vi "Sperre thrust alloc SF30K (SubVI) old.vi"(0 "Thruster rpms":dbl[](array[numeric]), 1 "manip14":u8, 2 "manip15":u8, 3 "manip16":u8, 5 "error in":errorcluster, 6 "dim 1+2":u8, 7 "Light 1":bool, 8 "dim 3+4":u8, 9 "Light 2":bool, 10 "digital2":u8, 11 "Light 3":bool, 12 "digital3":u8=2, 13 "Light 4":bool, 17 "HMI 1":bool, 18 "HMI 2":bool) -> (14 "telebuf":u8[](array[numeric]), 19 "error IO":errorcluster)   [LabVIEW 2011]
uses:
  <vilib>/imath/engines/lvmath2/RunTimeEngine/ErrorHandling/NIMS_Finalize Error.vi
  <vilib>/imath/engines/lvmath2/RunTimeEngine/BuiltInFunctions/uint8/NIMS_uint8(int).vi
  <instcachedir>/0/NIMS_uint8(int)_9D6EF81F86254677BB00410F9E5C6A1D.lvgen/NIMS_uint8(int)_9D6EF81F86254677BB00410F9E5C6A1D_000.vi
  <vilib>/imath/engines/lvmath2/RunTimeEngine/NodeEndStatement/NIMS_NodeEndStatement_Output.vi
  <instcachedir>/0/NIMS_NodeEndStatement_Output_53EC0D466D134D7ABD903AC30B43404B.lvgen/NIMS_NodeEndStatement_Output_53EC0D466D134D7ABD903AC30B43404B_016.vi
  <vilib>/imath/engines/lvmath2/RunTimeEngine/BuiltInFunctions/round/NIMS_round(DBL-S).vi
  <vilib>/imath/engines/lvmath2/RunTimeEngine/BuiltInFunctions/uint8/NIMS_uint8(real).vi
  <instcachedir>/0/NIMS_uint8(real)_CAA419FBB1354DA296C59E18C46DECF0.lvgen/NIMS_uint8(real)_CAA419FBB1354DA296C59E18C46DECF0_000.vi
  <instcachedir>/0/NIMS_uint8(int)_9D6EF81F86254677BB00410F9E5C6A1D.lvgen/NIMS_uint8(int)_9D6EF81F86254677BB00410F9E5C6A1D_001.vi
  <vilib>/imath/engines/lvmath2/RunTimeEngine/ReplaceToken/NIMS_Replace - Check Linear.vi
  <instcachedir>/0/NIMS_Replace - Check Linear_276AD648BD064726893CCF9ED6E2A728.lvgen/NIMS_Replace - Check Linear_276AD648BD064726893CCF9ED6E2A728_006.vi
  <vilib>/imath/engines/lvmath2/RunTimeEngine/ReplaceToken/NIMS_Replace - Size Check _(_)=S.vi
  <instcachedir>/0/NIMS_Replace - Size Check _(_)=S_9ABE7AF2D26C43EAA05192D5C1E6C624.lvgen/NIMS_Replace - Size Check _(_)=S_9ABE7AF2D26C43EAA05192D5C1E6C624_004.vi
  <vilib>/imath/engines/lvmath2/RunTimeEngine/ReplaceToken/NIMS_Replace - V(S)=S.vi
  <instcachedir>/0/NIMS_Replace - V(S)=S_16B13A4565AB46F59881314645612498.lvgen/NIMS_Replace - V(S)=S_16B13A4565AB46F59881314645612498_002.vi
  <vilib>/imathl/engines/lvmath/Functions/Error Handling/Create Error.vi
  <vilib>/imath/engines/lvmath2/RunTimeEngine/BuiltInFunctions/bitand/NIMS_bitand(SorS,SorS).vi
  <vilib>/imath/engines/lvmath2/RunTimeEngine/ErrorHandling/NIMS_Create Error From Enums.vi
  <vilib>/imath/engines/lvmath2/RunTimeEngine/VariableToken/Read/NIMS_Get Elements - CV(_) - Check.vi
  <instcachedir>/0/NIMS_Get Elements - CV(_) - Check_4CF014B95B49446692066C44E7C19A08.lvgen/NIMS_Get Elements - CV(_) - Check_4CF014B95B49446692066C44E7C19A08_006.vi
  <vilib>/imath/engines/lvmath2/RunTimeEngine/BuiltInFunctions/uint8/NIMS_uint8(uint).vi
  <instcachedir>/0/NIMS_uint8(uint)_4F8EF4DA29E74BF19348291C199FCD23.lvgen/NIMS_uint8(uint)_4F8EF4DA29E74BF19348291C199FCD23_002.vi
  <vilib>/imath/engines/lvmath2/RunTimeEngine/BuiltInFunctions/bitset/NIMS_bitset(RS,RS,RS).vi
  <vilib>/imath/engines/lvmath2/RunTimeEngine/BuiltInFunctions/bitget/NIMS_bitget(SorS,SorS).vi
  <instcachedir>/0/NIMS_uint8(uint)_4F8EF4DA29E74BF19348291C199FCD23.lvgen/NIMS_uint8(uint)_4F8EF4DA29E74BF19348291C199FCD23_001.vi
  <vilib>/imath/engines/lvmath2/RunTimeEngine/RangeToken/NIMS_Range_R2 - Integer.vi
  <instcachedir>/0/NIMS_Range_R2 - Integer_8B99B1FAA0BB43C693F13B8216F464EC.lvgen/NIMS_Range_R2 - Integer_8B99B1FAA0BB43C693F13B8216F464EC_000.vi
  <vilib>/imath/engines/lvmath2/RunTimeEngine/CommandStatement/MC_CommandStatement_break.vi
  <vilib>/imath/engines/lvmath2/RunTimeEngine/BuiltInFunctions/double/NIMS_double.vi
  <instcachedir>/0/NIMS_double_34E32F64C2B04A25A042F4CA881A0A41.lvgen/NIMS_double_34E32F64C2B04A25A042F4CA881A0A41_002.vi
  <vilib>/imath/engines/lvmath2/RunTimeEngine/BuiltInFunctions/mod/NIMS_mod_no_size_check.vi
  <instcachedir>/0/NIMS_mod_no_size_check_5393E3382FD241D281EEB71DA286C65B.lvgen/NIMS_mod_no_size_check_5393E3382FD241D281EEB71DA286C65B_008.vi
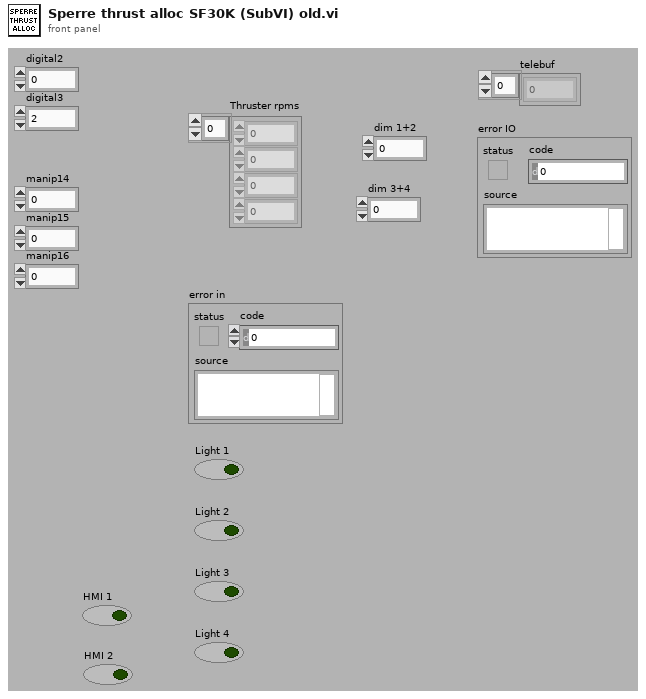
[diagram p1: front panel]
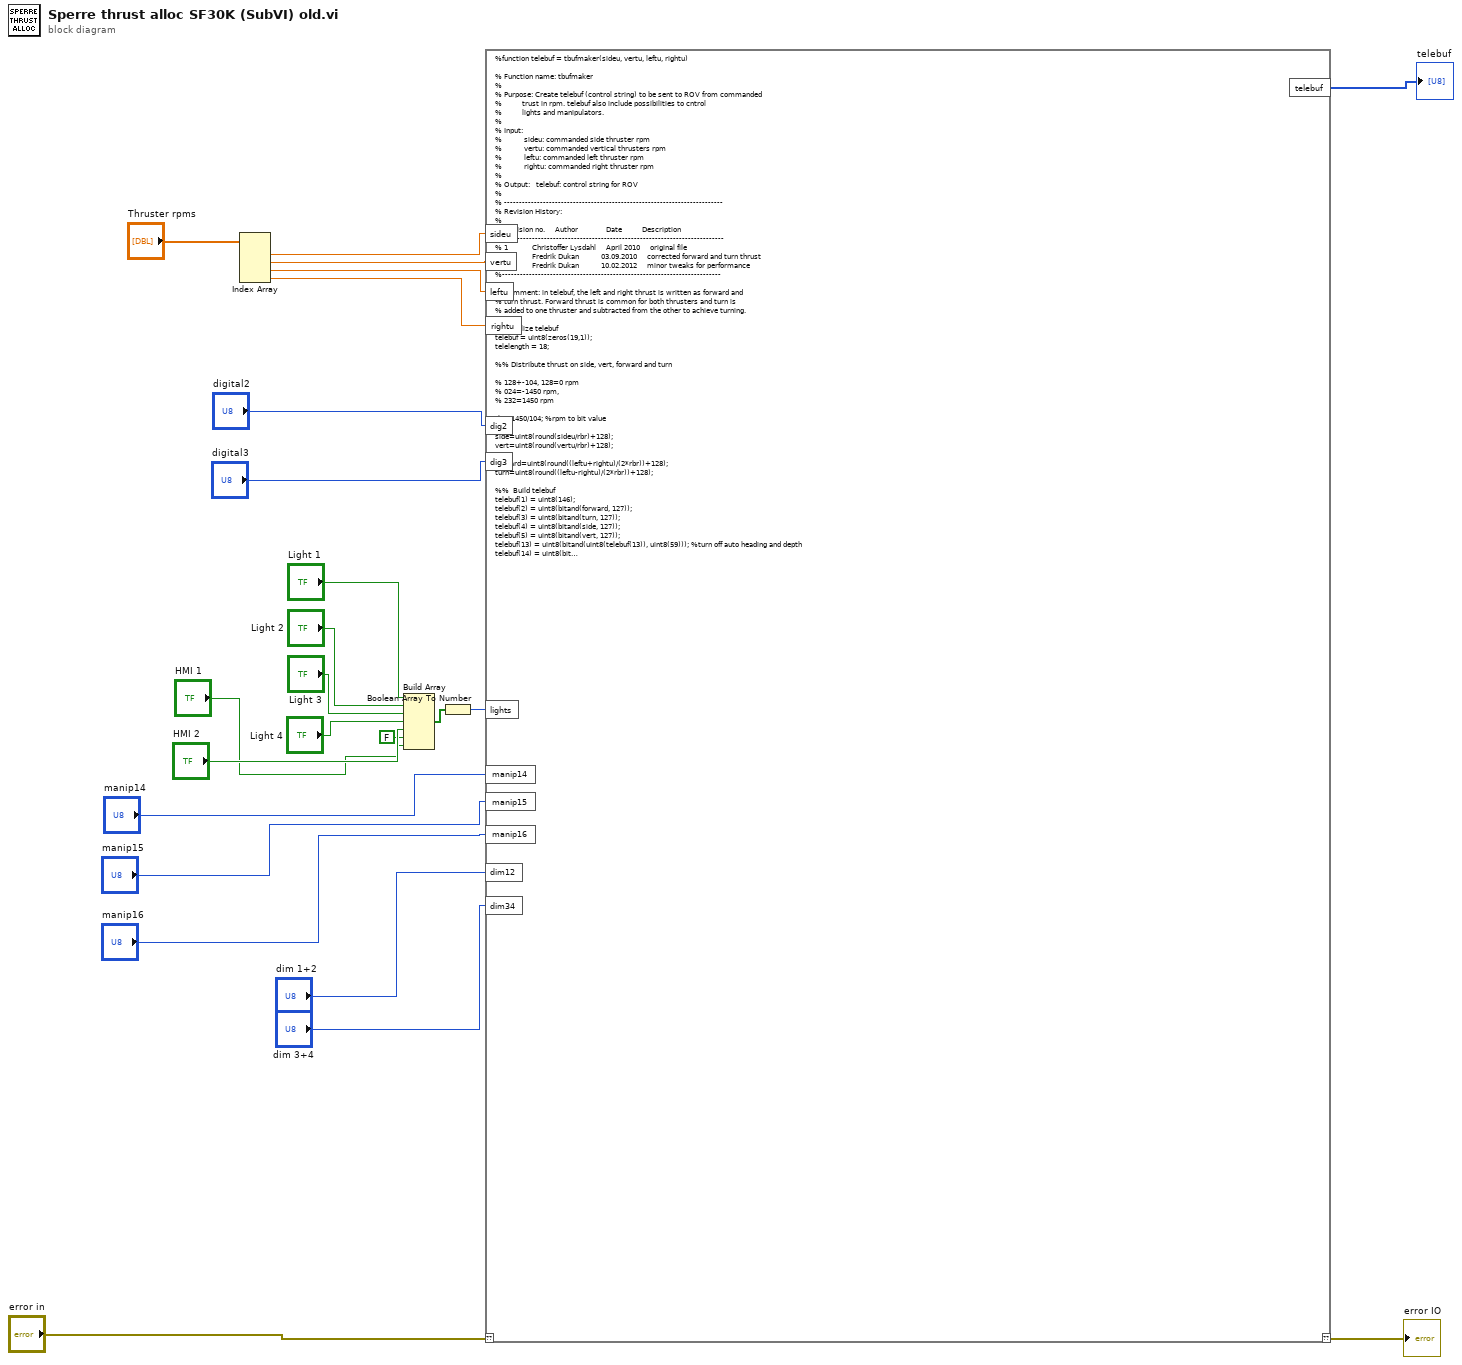
[diagram p0: block diagram]
diagram:
  n1 = Index Array(array="Thruster rpms") -> (element #1=w12:dbl, element #2=w11:dbl, element #3=w10:dbl, element #4=w9:dbl)  [unwired: 4 in]
  n2 = Build Array("Light 1", "Light 2", "Light 3", "Light 4", "HMI 2", FALSE ("element"), "HMI 1") -> (w21:bool[])
  n3 = Boolean Array To Number(Boolean array=w21) -> (number=w22:u32)
  n4 = mathscript code="%function telebuf = tbufmaker(sideu, vertu, leftu, rightu)\n\n% Function name: tbufmaker\n%\n% Purpose: Create telebuf (control string) to be sent to ROV from commanded\n%          trust in rpm. telebuf also include possibilities to cntrol\n%          lights and manipulators.\n%\n% Input:  \n%           sideu: commanded side thruster rpm\n%           vertu: commanded vertical thrusters rpm\n%           leftu: commanded left thruster rpm\n%           rightu: commanded right thruster rpm\n%\n% Output:   telebuf: control string for ROV\n%\n% -------------------------------------------------------------------------\n% Revision History:\n%\n% Revision no.     Author              Date          Description\n%--------------------------------------------------------------------------\n% 1            Christoffer Lysdahl     April 2010     original file\n% 2            Fredrik Dukan           03.09.2010     corrected forward and turn thrust\n% 3            Fredrik Dukan           10.02.2012     minor tweaks for performance \n%-------------------------------------------------------------------------\n\n% Comment: in telebuf, the left and right thrust is written as forward and\n% turn thrust. Forward thrust is common for both thrusters and turn is \n% added to one thruster and subtracted from the other to achieve turning.\n\n% Initialize telebuf\ntelebuf = uint8(zeros(19,1));\ntelelength = 18;\n\n%% Distribute thrust on side, vert, forward and turn\n\n% 128+-104, 128=0 rpm\n% 024=-1450 rpm,\n% 232=1450 rpm\n\nrbr=1450/104; %rpm to bit value\n\nside=uint8(round(sideu/rbr)+128);\nvert=uint8(round(vertu/rbr)+128);\n\nforward=uint8(round((leftu+rightu)/(2*rbr))+128);\nturn=uint8(round((leftu-rightu)/(2*rbr))+128);\n\n%%  Build telebuf\ntelebuf(1) = uint8(146);\ntelebuf(2) = uint8(bitand(forward, 127));\ntelebuf(3) = uint8(bitand(turn, 127));\ntelebuf(4) = uint8(bitand(side, 127));\ntelebuf(5) = uint8(bitand(vert, 127));\ntelebuf(13) = uint8(bitand(uint8(telebuf(13)), uint8(59))); %turn off auto heading and depth\ntelebuf(14) = uint8(bitset(uint8(telebuf(14)), 7, 0)); % note: not needed in matlab\ntelebuf(14) = uint8(bitset(uint8(telebuf(14)), 7, bitget(forward, 8)));\ntelebuf(14) = uint8(bitset(uint8(telebuf(14)), 6, 0)); % note: not needed in matlab\ntelebuf(14) = uint8(bitset(uint8(telebuf(14)), 6, bitget(turn, 8)));\ntelebuf(14) = uint8(bitset(uint8(telebuf(14)), 5, 0)); % note: not needed in matlab\ntelebuf(14) = uint8(bitset(uint8(telebuf(14)), 5, bitget(side, 8)));\ntelebuf(14) = uint8(bitset(uint8(telebuf(14)), 4, 0)); % note: not needed in matlab\ntelebuf(14) = uint8(bitset(uint8(telebuf(14)), 4, bitget(vert, 8)));\n\n%lights on\ntelebuf(7) = dim12;\ntelebuf(8) = dim34;\ntelebuf(9) = uint8(127);\ntelebuf(10) =uint8(lights);\ntelebuf(11) =dig2;\ntelebuf(12) =dig3;\ntelebuf(15) = manip14;\ntelebuf(16) = manip15;\ntelebuf(17) = manip16;\n\n%checksums\nchk = uint8(0);\n\nfor i = 1:telelength - 1\n    chk = chk + telebuf(i);\nend\nchk1 = double(chk);\ncheck1 = uint8(bitand(uint8(floor(chk1/256)), 127));\ncheck2 = uint8(bitand(mod(chk, 256) , 127));\ntelebuf(18) = check1;\ntelebuf(19) = check2;"("??"="error in", "sideu"=w12, "vertu"=w11, "leftu"=w10, "rightu"=w9, "dim12"="dim 1+2", "dim34"="dim 3+4", "lights"=w22, "manip14"="manip14", "manip15"="manip15", "manip16"="manip16", "dig2"="digital2", "dig3"="digital3") -> ("??"=→"error IO":errorcluster, "telebuf"=→"telebuf":u8[])
